vi "K6514_ReadCurrentOnly.vi"(7 "error in (no error)":errorcluster, 10 "VISA resource name":refnum<visa-resource-name>) -> (0 "error out":errorcluster, 1 "Response":string, 2 "Current (A)":dbl, 3 "VISA resource name out":refnum<visa-resource-name>)   [LabVIEW 2024]
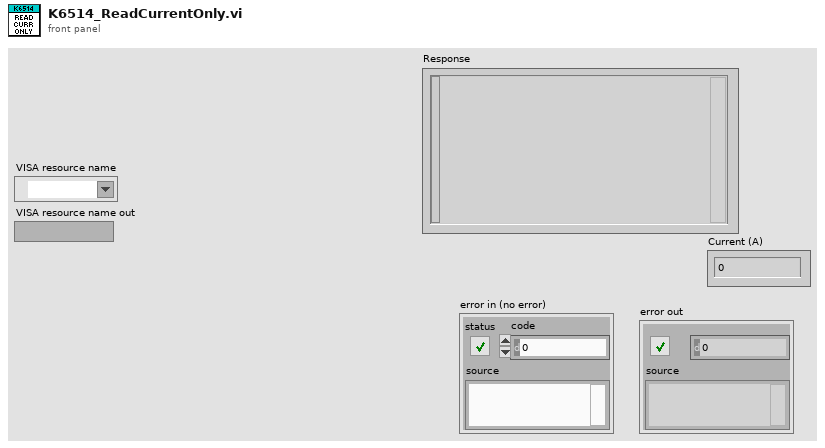
[diagram p1: front panel]
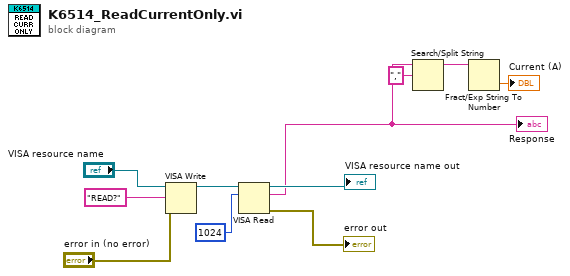
[diagram p0: block diagram]
diagram:
  n1 = VISA Write(VISA resource name="VISA resource name", write buffer="READ?" ("String"), error in (no error)="error in (no error)") -> (VISA resource name out=w8:refnum<visa-resource-name>)  [unwired: 2 out]
  n2 = VISA Read(VISA resource name=w8, byte count=u32 1024 ("Read Count")) -> (VISA resource name out=→"VISA resource name out":refnum<visa-resource-name>, read buffer=w1:string, error out=→"error out":errorcluster)  [unwired: 1 in, 1 out]
  "Response" <- w1
  n3 = Search/Split String(string=w1, search string/char (-)=",") -> (substring before match=w6:string)  [unwired: 1 in, 2 out]
  n4 = Fract/Exp String To Number(string=w6) -> (number=→"Current (A)":dbl)  [unwired: 3 in, 1 out]
